vi "Get Driver Version.vi"(8 "error in (no error)":errorcluster, 11 "TDCManager":T1) -> (0 "error out":errorcluster, 2 "Driver Version":i32, 3 "TDCManager":T1)   [LabVIEW 2016, in "HPTDC Driver Library.lvlib"]
uses:
  HPTDC Driver Library.lvlib
  Typedefs/TDCManager.ctl
  C:/Users/CRT Controller/CRTC Labview Application/Source/HPTDC Driver Library Folder/Library files/hptdc_net4_3.7.0_x64.dll
  hptdc_net4_3.7.0_x64.dll
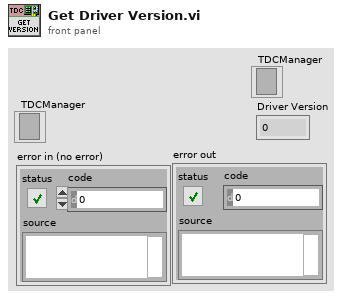
[diagram p1: front panel]
types:
  T1 = typedef "HPTDC Driver Library.lvlib/TDCManager.ctl" = refnum<k24>
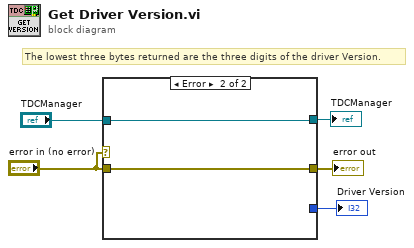
[diagram p0: block diagram]
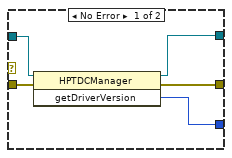
[diagram p2: hidden frame]
diagram:
  # "The lowest three bytes returned are the three digits of the driver Version."
  n1 = case shown="Error" "error in (no error)" {
    tunnel: "error in (no error)" -> [w10 w11]
    tunnel: [w9 w11] -> w5
    tunnel: [w8 w12] -> w4
    tunnel: "TDCManager" -> [w7 w12]
    tunnel: [w6 _] -> w2
    frame No Error {
      n2 = invoke class="HPTDCManager" method="getDriverVersion"(reference=w7, error in=w10) -> (reference out=w8:T1, error out=w9:errorcluster, "getDriverVersion"=w6:i32)  [unwired: 1 in]
    }
    frame Error {
    }
  }
  "error out" <- w5
  "TDCManager" <- w4
  "Driver Version" <- w2
